vi "Disconnect.vi"(8 "error in (no error)":errorcluster, 11 "Smart_Eye_Pro_Driver in":refnum<class "SmartEyeProDriver.lvclass">) -> (0 "error out":errorcluster, 3 "Smart_Eye_Pro_Driver out":refnum<class "SmartEyeProDriver.lvclass">)   [LabVIEW 2020, in "SmartEyeProDriver.lvclass"]
uses:
  SmartEyeProDriver.lvclass
  SmartEyeProDriver.lvclass/SmartEyeProDriver.ctl
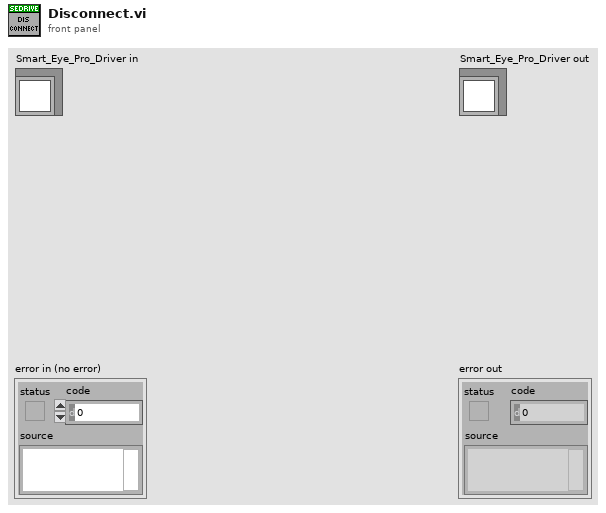
[diagram p1: front panel]
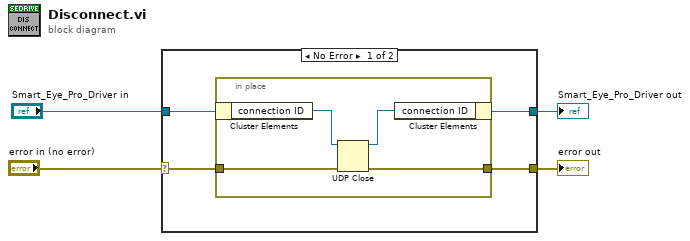
[diagram p0: block diagram]
diagram:
  n1 = case shown="No Error" "error in (no error)" {
    selector: "error in (no error)" -> [w7 w14]
    tunnel: [w6 w14] -> w3
    tunnel: [w5 w13] -> w1
    tunnel: "Smart_Eye_Pro_Driver in" -> [w8 w13]
    frame No Error {
      n2 = in-place {
        in-place-border: w7 -> [w12]
        in-place-border: [w11] -> w6
        n3 = in-place-cluster #1(w8) -> ("connection ID"=w10:refnum<k16>)
        n4 = UDP Close(connection ID=w10, 8:w12) -> (connection ID out=w9:refnum<k16>, error out=w11:errorcluster)
        n5 = in-place-cluster #1("connection ID"=w9) -> (w5:refnum<class "SmartEyeProDriver.lvclass">)
      }
    }
    frame Error {
    }
  }
  "error out" <- w3
  "Smart_Eye_Pro_Driver out" <- w1
